vi "Write TCP Stream.vi"(8 "error in (no error)":errorcluster, 9 "timeout (ms)":i32=200, 10 "Data":u8[](array[numeric]), 11 "TCP_Streamer in":refnum<class "TCP_Streamer_Publisher.lvclass">=refnum) -> (0 "error out":errorcluster, 2 "Timeout":bool, 3 "TCP_Streamer out":refnum<class "TCP_Streamer_Publisher.lvclass">)   [LabVIEW 2021, in "TCP_Streamer_Publisher.lvclass"]
doc: "Some TCP streaming applications don't want a long timeout for the TCP write as that may cause the application to become unresponsive if the receiving application is not accepting data fast enough.\nIf the TCP buffer on sender or receiver is full and we timeout, the TCP write may send a partial message. This can cause data corruption for data streaming applications. For a lossless stream we need to complete sending the reset of the message \n\nThis will check if all the data was sent.\nIf not all data was sent, it will set a timeout and update an offset. \nIt is expected the calling application will respond to the timeout and try to resend the exact same message.\nOn the next call it will only write the remaining bytes of the message so an complete message is eventually sent."
uses:
  TCP_Streamer_Publisher.lvclass
  Typedef/State.ctl
  TCP_Streamer_Publisher.lvclass/TCP_Streamer_Publisher.ctl
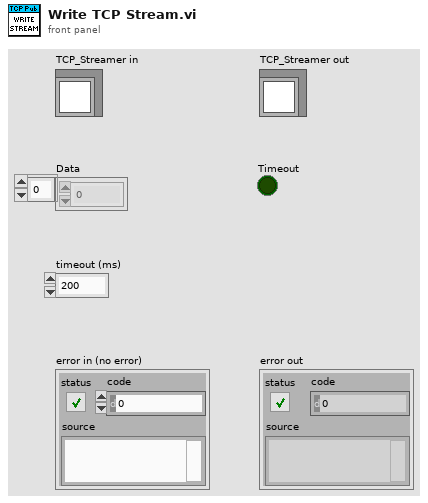
[diagram p1: front panel]
types:
  T1 = typedef "TCP_Streamer_Publisher.lvclass/State.ctl" = enum16{"Stopped", "Listening", "Ready for Data", "Ready to Send", "Sending"}
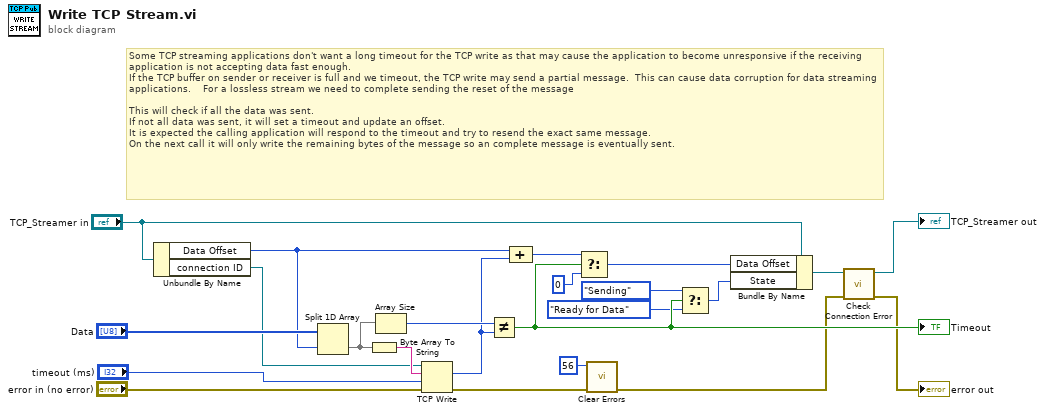
[diagram p0: block diagram]
diagram:
  # "Some TCP streaming applications don't want a long timeout for the TCP write as that may cause the application to become unresponsive if the receiving application is not accepting data fast enough.\nIf the TCP buffer on sender or receiver is full and we timeout, the TCP write may send a partial message.  This can cause data corruption for data streaming applications.    For a lossless stream we need to complete sending the reset of the message \n\nThis will check if all the data was sent.\nIf not all data was sent, it will set a timeout and update an offset.  \nIt is expected the calling application will respond to the timeout and try to resend the exact same message.\nOn the next call it will only write the remaining bytes of the message so an complete message is eventually sent."
  n1 = Unbundle By Name("TCP_Streamer in") -> ("Data Offset"=w12:i32, "connection ID"=w11:refnum<k5>)
  n2 = Split 1D Array(array="Data", index=w12) -> (second subarray=w17:u8[])  [unwired: 1 out]
  n3 = Byte Array To String(unsigned byte array=w17) -> (string=w21:string)
  n4 = Array Size(array=w17) -> (size(s)=w16:i32)
  n5 = TCP Write(connection ID=w11, data in=w21, error in (no error)="error in (no error)", 9:"timeout (ms)") -> (bytes written=w14:i32, error out=w19:errorcluster)  [unwired: 1 out]
  n6 = Not Equal?(x=w16, y=w14) -> (x != y?=w8:bool)
  "Timeout" <- w8
  n7 = Compound Arithmetic op=ADD(w12, w14) -> (w15:i32)
  n8 = Select(t=w15, s=w8, f=0) -> (s? t:f=w9:i32)
  n9 = call <vilib>:"Clear Errors.vi"("error in (no error)"=w19, "specific error code to clear (0: all)"=56) -> ("error out"=w4:errorcluster)  [unwired: 4 in, 1 out]
  n10 = Select(t=State."Sending" ("State"), s=w8, f=State."Ready for Data" ("State")) -> (s? t:f=w7:T1)
  n11 = Bundle By Name(cluster="TCP_Streamer in", "Data Offset"=w9, "State"=w7) -> (w3:refnum<class "TCP_Streamer_Publisher.lvclass">)
  n12 = call "Check Connection Error.vi"("error in (no error)"=w4, "TCP_Streamer_Publisher in"=w3) -> ("error out"=→"error out":errorcluster, "TCP_Streamer_Publisher out"=→"TCP_Streamer out":refnum<class "TCP_Streamer_Publisher.lvclass">)  [unwired: 8 in]
